vi "Send tt20panel_DO_stream_data.vi"(6 "Overwrite?":bool, 7 "Message Priority (Normal)":T2=enum."Normal", 8 "error in (no error)":errorcluster, 9 "stream_settings":T1, 10 "stop_counts":refnum<queue>, 11 "Message Enqueuer":refnum<class "Message Enqueuer.lvclass">) -> (0 "error out":errorcluster, 3 "Message Enqueuer out":refnum<class "Message Enqueuer.lvclass">)   [LabVIEW 2015, in "tt20panel_DO_stream_data Msg.lvclass"]
doc: "This VI sends the message to an actor."
uses:
  tt20panel_DO_stream_data Msg.lvclass
  <vilib>/ActorFramework/Message Enqueuer/Message Enqueuer.lvclass
  <vilib>/ActorFramework/Message Enqueuer/Message Priority.ctl
  tt20panel_class/tt20_stream_settings_tdef.ctl
  tt20panel_DO_stream_data Msg.lvclass/tt20panel_DO_stream_data Msg.ctl
  <vilib>/ActorFramework/Message Enqueuer/Message Enqueuer.lvclass/Message Enqueuer.ctl
  <vilib>/ActorFramework/Message Priority Queue/Priority Enqueue.vi
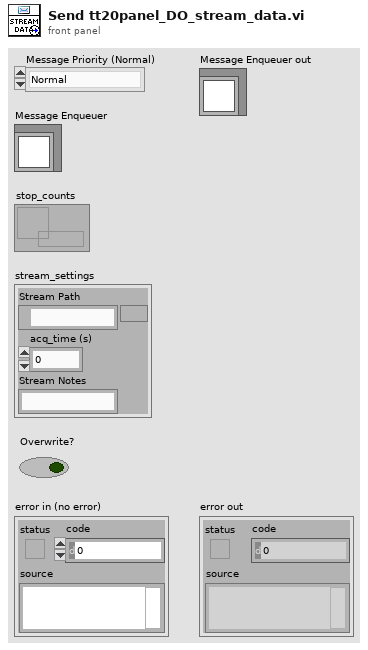
[diagram p1: front panel]
types:
  T1 = typedef "tt20_stream_settings_tdef.ctl" = cluster{"Stream Path":path, "acq_time (s)":u32, "Stream Notes":string}
  T2 = typedef "Actor Framework.lvlib/Message Enqueuer.lvclass/Message Priority.ctl" = enum16{"Low", "Normal", "High"}
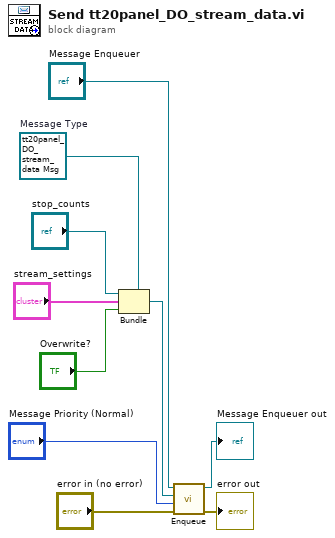
[diagram p0: block diagram]
diagram:
  w7 = refnum<class "tt20panel_DO_stream_data Msg.lvclass"> refnum  # Message Type
  n1 = Bundle(cluster=w7, "stop_counts", "stream_settings", "Overwrite?") -> (w6:refnum<class "tt20panel_DO_stream_data Msg.lvclass">)
  n2 = call <vilib>:"Enqueue.vi"("error in (no error)"="error in (no error)", "Message Priority (Normal)"="Message Priority (Normal)", "Message"=w6, "Message Enqueuer in"="Message Enqueuer") -> ("error out"=→"error out":errorcluster, "Message Enqueuer out"=→"Message Enqueuer out":refnum<class "Message Enqueuer.lvclass">)  [unwired: 6 in]
